vi "get_mcs_data2.vi"(10 "MCS Parameters":T1={"Scan Length (Bins)"=64.0, "Dwell Time (s)"=1e-07, "Gate Channel Settings"={"Threshold (V)"=0.0, "Edge"=enum."Falling", "Input Impedence"=enum."1k Ohm"}, "Trig Channel Settings"={"Threshold (V)"=0.0, "Edge"=enum."Falling", "Input Impedence"=enum."1k Ohm"}, "Input 1 Settings"={"Threshold (V)"=0.0, "Edge"=enum."Falling", "Input Impedence"=enum."1k Ohm"}, "Input 2 Settings"={"Threshold (V)"=0.0, "Edge"=enum."Falling", "Input Impedence"=enum."1k Ohm"}, "Number of Sweeps"=0, "Number of Sequential Cycles"=0.0, "Number of Sequences"=0.0, "Sweep Preset"=FALSE, "Sequential Mode"=FALSE, "DAC 1 Ramp Settings"={"Ramp Mode"=enum."Fixed", "Ramp Start Value (V)"=0.0, "Ramp Length (Steps)"=1, "Step Width (bins)"=0, "Step Size (V)"=0.0}, "DAC 2 Output (V)"=0.0, "SYNC Output"=enum."40 MHz Clock", "ROI Min"=0, "ROI Max"=1, "Dual MCS Mode"=FALSE, "DAC 2 Toggle"=FALSE, "MCS on/off"=FALSE, "ROI Max 2"=1, "ROI Min 2"=0, "Sum ROI Only"=FALSE, "Use ROI For \nEach Loop"=FALSE} {"ROI Max 2" min=1; "ROI Min 2" min=0; "ROI Max" min=1; "ROI Min" min=0; "DAC 2 Output (V)" min=-10.0 max=10.0 step=0.00488; "DAC 1 Ramp Settings"."Step Size (V)" min=0.0 max=10.0 step=0.00244 format="%#_4g"; "DAC 1 Ramp Settings"."Step Width (bins)" min=1; "DAC 1 Ramp Settings"."Ramp Length (Steps)" min=1; "DAC 1 Ramp Settings"."Ramp Start Value (V)" min=0.0 max=10.0 step=0.00244; "Number of Sweeps" min=0 format="%.0p"; "Input 2 Settings"."Threshold (V)" min=-2.5 max=2.5 step=0.001; "Input 1 Settings"."Threshold (V)" min=-2.5 max=2.5 step=0.001; "Trig Channel Settings"."Threshold (V)" min=-2.5 max=2.5 step=0.001; "Gate Channel Settings"."Threshold (V)" min=-2.5 max=2.5 step=0.001; "Dwell Time (s)" min=1e-07 step=2.5e-08 format="%#_6p"; "Scan Length (Bins)" min=64.0 max=524288.0 format="%#_7f"}) -> (2 "2d Data":u32[][](array[numeric]))   [LabVIEW 2015]
uses:
  Controls/MCS/mcs_control_panel.ctl
  Controls/MCS/mcs_channel.ctl
  Controls/MCS/ramp_control.ctl
panel:
  in  "Wait until next time":u32
  out "Sweeps":dbl(graph)
  out "Waveform Graph":u32[](graph)
  out "Response":string
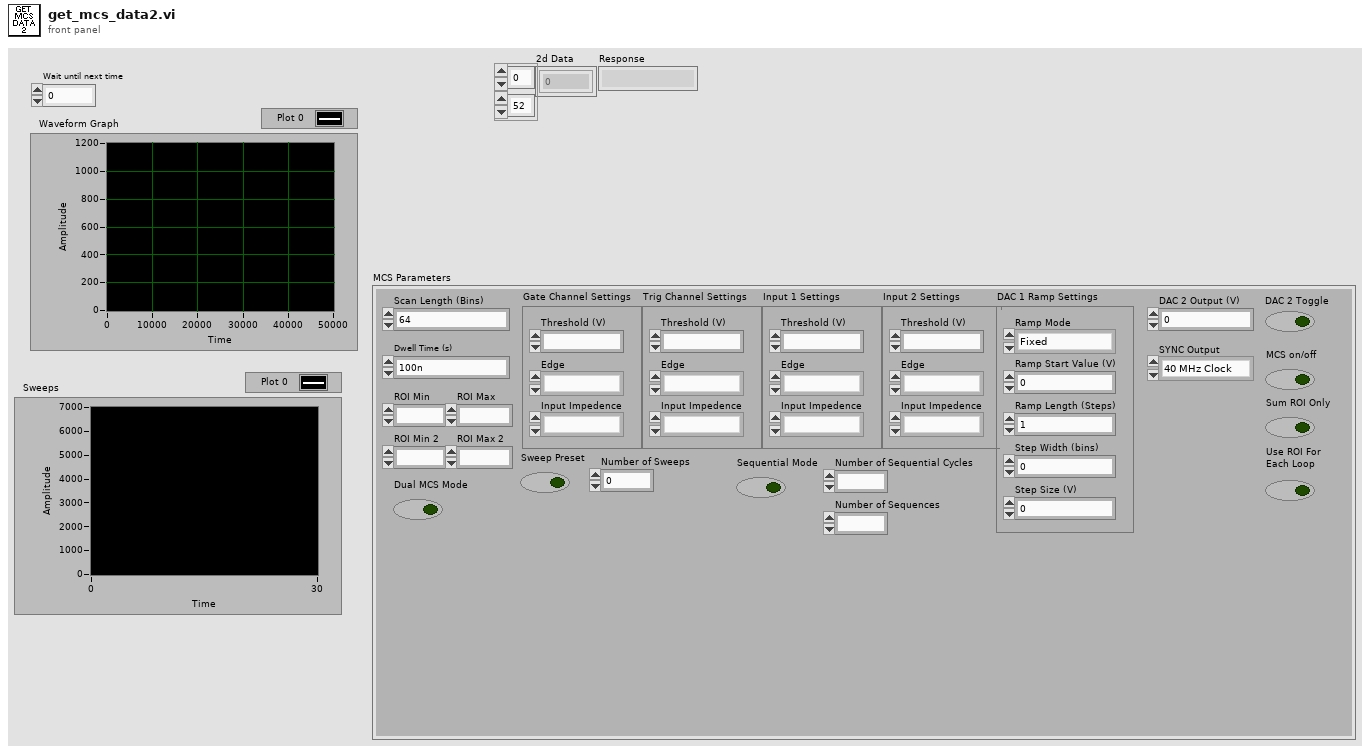
[diagram p1: front panel]
types:
  T1 = typedef "mcs_control_panel.ctl" = cluster{"Scan Length (Bins)":dbl, "Dwell Time (s)":dbl, "Gate Channel Settings":T2, "Trig Channel Settings":T2, "Input 1 Settings":T2, "Input 2 Settings":T2, "Number of Sweeps":i32, "Number of Sequential Cycles":dbl, "Number of Sequences":dbl, "Sweep Preset":bool, "Sequential Mode":bool, "DAC 1 Ramp Settings":T3, "DAC 2 Output (V)":dbl, "SYNC Output":enum16{"40 MHz Clock", "Gate Disc Signal", "Trigger Disc Signal", "Counter 1 Disc Signal", "Counter 2 Disc Signal", "Definitely Not Used", "Not Used", "1 kHz Signal", "Also Not Used", "MCS On/Off", "End of Time Bin", "Ramp Increment Trig", "Step Count Trigger", "'GO'-Line", "Ramp Down Trigger", "Logic 1"}, "ROI Min":i32, "ROI Max":i32, "Dual MCS Mode":bool, "DAC 2 Toggle":bool, "MCS on/off":bool, "ROI Max 2":i32, "ROI Min 2":i32, "Sum ROI Only":bool, "Use ROI For \nEach Loop":bool}
  T2 = typedef "mcs_channel.ctl" = cluster{"Threshold (V)":dbl, "Edge":enum16{"Falling", "Rising"}, "Input Impedence":enum16{"1k Ohm", "50 Ohm"}}
  T3 = typedef "ramp_control.ctl" = cluster{"Ramp Mode":enum16{"Fixed", "Triangle", "Sawtooth"}, "Ramp Start Value (V)":dbl, "Ramp Length (Steps)":i32, "Step Width (bins)":i32, "Step Size (V)":dbl}
  T4 = cluster{"Running":i32, "Dummy1":i32, "Realtime":dbl, "TotalSum":dbl, "RoiSum":dbl, "TotalRate":dbl, "NetSum":dbl, "Livetime(Sweeps)":dbl, "Deadtime":dbl, "Maxval":u32, "Dummy2":i32}
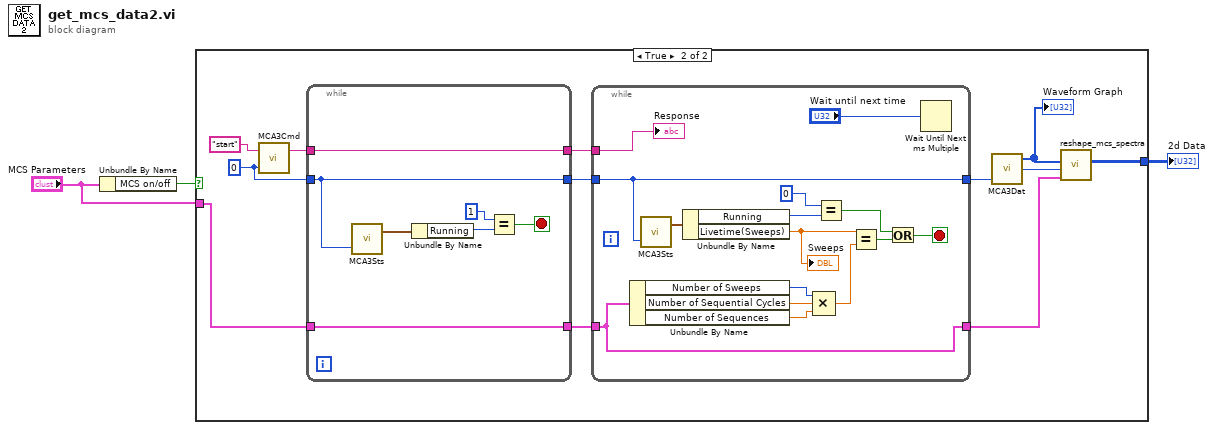
[diagram p0: block diagram]
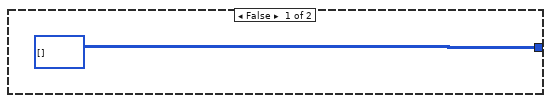
[diagram p2: hidden frame]
diagram:
  n1 = Unbundle By Name("MCS Parameters") -> ("MCS on/off"=w3:bool)
  n2 = case shown="True" w3 {
    tunnel: "MCS Parameters" -> [_ w10]
    tunnel: [u32[][] [] ("2d Data") w15] -> w1
    frame False {
    }
    frame True {
      w6 = 0 ("MCA #")
      n3 = call "MCA3Cmd.vi"("MCA #"=w6, "Command"="start") -> ("Response"=w8:string)  [unwired: 1 in]
      n4 = while {
        tunnel: w10 -> [w23]
        tunnel: [w23] -> w9
        tunnel: w8 -> [w17]
        tunnel: [w17] -> w7
        tunnel: w6 -> [w22]
        tunnel: [w22] -> w5
        stop <- w18 stop-if-true
        n5 = call "MCA3Sts.vi"("MCD #"=w22) -> ("MCA-3 Status"=w21:T4)  [unwired: 1 in, 1 out]
        n6 = Unbundle By Name(w21) -> ("Running"=w20:i32)
        n7 = Equal?(x=1, y=w20) -> (x = y?=w18:bool)
      }
      n8 = while {
        tunnel: w7 -> [w37]
        tunnel: w5 -> [w31]
        tunnel: [w36] -> w14
        tunnel: w9 -> [w36]
        tunnel: [w31] -> w13
        stop <- w26 stop-if-true
        n9 = Unbundle By Name(w36) -> ("Number of Sweeps"=w33:i32, "Number of Sequential Cycles"=w34:dbl, "Number of Sequences"=w35:dbl)
        n10 = call "MCA3Sts.vi"("MCD #"=w31) -> ("MCA-3 Status"=w38:T4)  [unwired: 1 in, 1 out]
        n11 = Unbundle By Name(w38) -> ("Running"=w29:i32, "Livetime(Sweeps)"=w25:dbl)
        "Sweeps" <- w25
        n12 = Compound Arithmetic op=MULTIPLY(w33, w34, w35) -> (w32:dbl)
        n13 = Equal?(x=0, y=w29) -> (x = y?=w27:bool)
        n14 = Equal?(x=w25, y=w32) -> (x = y?=w30:bool)
        n15 = Or(x=w27, y=w30) -> (x .or. y?=w26:bool)
        n16 = Wait Until Next ms Multiple(millisecond multiple="Wait until next time") -> ()  [unwired: 1 out]
        "Response" <- w37
      }
      n17 = call "MCA3Dat.vi"("MCD #"=w13) -> ("Spectrum Length"=w12:i32, "Data"=w11:u32[])  [unwired: 2 in, 1 out]
      "Waveform Graph" <- w11
      n18 = call "reshape_mcs_spectra.vi"("MCS Parameters"=w14, "Spectrum Length"=w12, "Data"=w11) -> ("2d Data"=w15:u32[][])  [unwired: 8 in]
    }
  }
  "2d Data" <- w1
